vi "niScope Configure Trigger (poly).vi"   [LabVIEW 2013]
doc: "Configures the digitizer for different types of triggering."
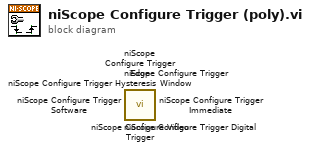
[diagram p0: block diagram]
diagram:
  n1 = call <instrlib>:"niScope Configure Video Trigger.vi"() -> ()  [unwired: 14 in, 2 out]
  n2 = call <instrlib>:"niScope Configure Trigger Window.vi"() -> ()  [unwired: 14 in, 2 out]
  n3 = call <instrlib>:"niScope Configure Trigger Software.vi"() -> ()  [unwired: 14 in, 2 out]
  n4 = call <instrlib>:"niScope Configure Trigger Immediate.vi"() -> ()  [unwired: 14 in, 2 out]
  n5 = call <instrlib>:"niScope Configure Trigger Hysteresis.vi"() -> ()  [unwired: 14 in, 2 out]
  n6 = call <instrlib>:"niScope Configure Trigger Edge.vi"() -> ()  [unwired: 14 in, 2 out]
  n7 = call <instrlib>:"niScope Configure Trigger Digital.vi"() -> ()  [unwired: 14 in, 2 out]
